vi "Vision Processing.vi"(4 "error in (no error)":errorcluster) -> ()   [LabVIEW 2016]
doc: "This VI runs in parallel to other tasks. It gets images from the camera, processes them for color or shape and use that information to affect robot behavior."
uses:
  Robot Global Data.vi
  Target x Location.vi
panel:
  out "Image":T1(plugin-control)
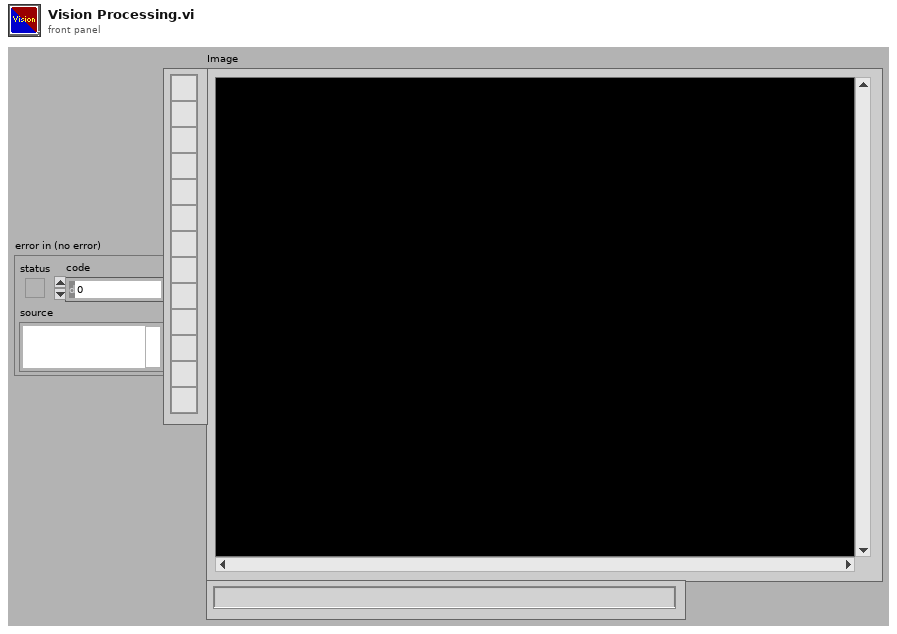
[diagram p1: front panel]
types:
  T1 = typedef "IMAQ Image.ctl" = refnum<image>
  T2 = typedef "Image Type" = u32
  T3 = typedef "WPI_CameraDevRef.ctl" = cluster{"Camera Address":string, "CameraStatus":errorcluster}
  T4 = cluster{"Global Rectangle":cluster{"x1Left":i32, "y1Top":i32, "x2Right":i32, "y2Bottom":i32}, "Centroid":cluster{"x":sgl, "y":sgl}, "Object Size":u32, "Score":dbl}[]
  T5 = typedef "WPI_CameraImageSize.ctl" = enum16{"640x480", "320x240", "160x120", "Custom"}
  T6 = cluster{"Global Rectangle":cluster{"x1Left":i32, "y1Top":i32, "x2Right":i32, "y2Bottom":i32}, "Centroid":cluster{"x":sgl, "y":sgl}, "Object Size":u32, "Score":dbl}
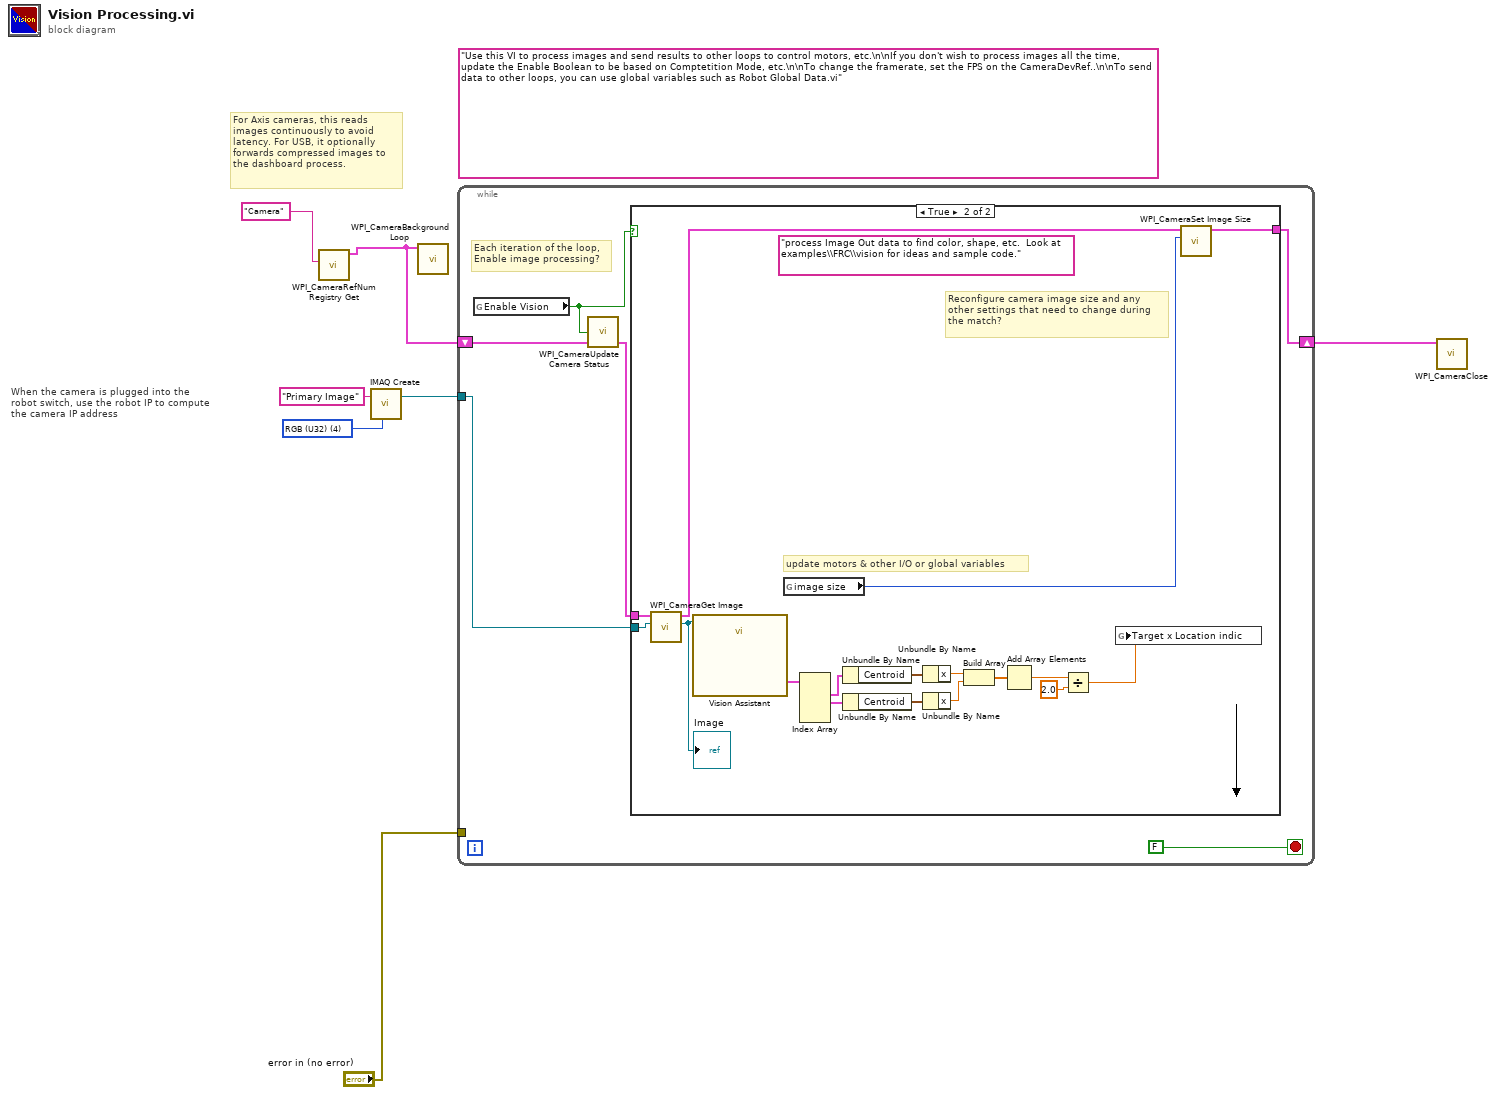
[diagram p0: block diagram]
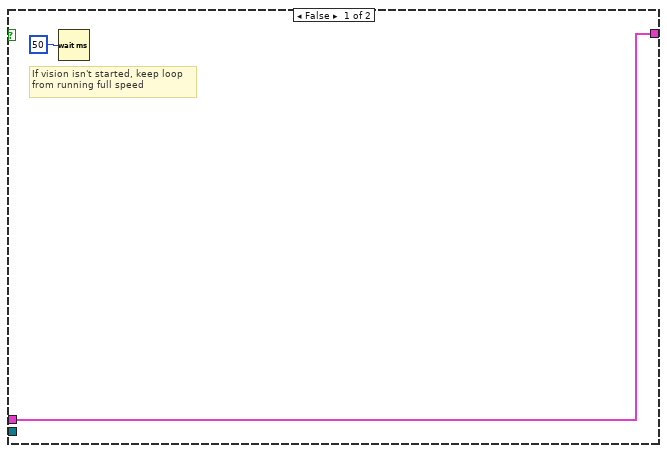
[diagram p2: hidden frame]
diagram:
  (unwired) "Use this VI to process images and send results to other loops to control motors, etc.\n\nIf you don't wish to process images all the time, update the Enable Boolean to be based on Comptetition Mode, etc.\n\nTo change the framerate, set the FPS on the CameraDevRef..\n\nTo send data to other loops, you can use global variables such as Robot Global Data.vi"
  w7 = T2 4 items=["Grayscale (U8)", "Grayscale (I16)", "Grayscale (SGL)", "Complex (CSG)", "RGB (U32)", "HSL (U32)", "RGB (U64)"] ("Image Type")
  # "When the camera is plugged into the\nrobot switch, use the robot IP to compute\nthe camera IP address"
  # "For Axis cameras, this reads\nimages continuously to avoid\nlatency. For USB, it optionally\nforwards compressed images to\nthe dashboard process."
  n1 = call <vilib>:"WPI_CameraRefNum Registry Get.vi"("refnum name"="Camera") -> ("CameraDevRef"=w2:T3)  [unwired: 9 in, 1 out]
  n2 = call "IMAQ Create"("Image Name"="Primary Image", "Image Type"=w7) -> ("New Image"=w5:T1)  [unwired: 2 in, 2 out]
  n3 = call <vilib>:"WPI_CameraBackground Loop.vi"("CameraDevRef"=w2) -> ()  [unwired: 11 in]
  n4 = while {
    shift-right: [w12] -> w4
    shift-left: w2 -> [w10]
    tunnel: w5 -> [w11]
    tunnel: "error in (no error)" -> [_]
    stop <- FALSE stop-if-true
    # "Each iteration of the loop,\nEnable image processing?"
    n5 = global read "Robot Global Data.vi" "Enable Vision"() -> (w8:bool)
    n6 = call <vilib>:"WPI_CameraUpdate Camera Status.vi"("CameraDevRef In"=w10, "Enable Vision"=w8) -> ("CameraDevRef Out"=w9:T3)  [unwired: 3 in]
    n7 = case shown="True" w8 {
      tunnel: w11 -> [_ w31]
      tunnel: [w15 w32] -> w12
      tunnel: w9 -> [w15 w29]
      frame False {
        # "If vision isn't started, keep loop\nfrom running full speed"
        n8 = Wait (ms)(milliseconds to wait=u32 50) -> ()  [unwired: 1 out]
      }
      frame True {
        (unwired) "process Image Out data to find color, shape, etc.  Look at examples\\FRC\\vision for ideas and sample code."
        # "update motors & other I/O or global variables"
        # "Reconfigure camera image size and any\nother settings that need to change during\nthe match?"
        n9 = call <vilib>:"WPI_CameraGet Image.vi"("Image"=w31, "CameraDevRef"=w29) -> ("Image Out"=w18:T1, "CameraDevRef Out"=w28:T3)  [unwired: 1 in, 7 out]
        "Image" <- w18
        n10 = call "Vision Assistant"("Image In"=w18) -> ("Shape Report (Shape Matching 1)"=w17:T4)  [unwired: 24 in, 2 out]
        n11 = global read "Robot Global Data.vi" "image size"() -> (w30:T5)
        n12 = Index Array(array=w17) -> (element #1=w27:T6, element #2=w25:T6)  [unwired: 4 in, 2 out]
        n13 = Unbundle By Name(w27) -> ("Centroid"=w26:cluster{"x":sgl, "y":sgl})
        n14 = Unbundle By Name(w25) -> ("Centroid"=w24:cluster{"x":sgl, "y":sgl})
        n15 = Unbundle By Name(w26) -> ("x"=w23:sgl)
        n16 = Unbundle By Name(w24) -> ("x"=w22:sgl)
        n17 = Build Array(w23, w22) -> (w21:sgl[])
        n18 = Add Array Elements(numeric array=w21) -> (sum=w20:sgl)
        n19 = Divide(x=w20, y=sgl 2.0) -> (x/y=w16:sgl)
        n20 = global write "Target x Location.vi" "Target x Location indic"(w16) -> ()
        n21 = call <vilib>:"WPI_CameraSet Image Size.vi"("Image Size"=w30, "CameraDevRef"=w28) -> ("CameraDevRef Out"=w32:T3)  [unwired: 2 in, 7 out]
      }
    }
  }
  n22 = call <vilib>:"WPI_CameraClose.vi"("CameraDevRef"=w4) -> ()  [unwired: 1 in, 10 out]
